vi "YTicks0003.vi"   [LabVIEW 2013]
uses:
  <vilib>/Heliosphere Research LLC/Advanced Plotting Toolkit/api_core/NewPlotType.ctl
  <vilib>/Heliosphere Research LLC/Advanced Plotting Toolkit/Advanced Plotting Toolkit.lvlib
types:
  T1 = typedef "Advanced Plotting Toolkit.lvlib/NewPlotType.ctl" = enum16{"Rectangular Axes", "Polar Axes"}
  T2 = typedef "Advanced Plotting Toolkit.lvlib/PlotID.ctl" = i32
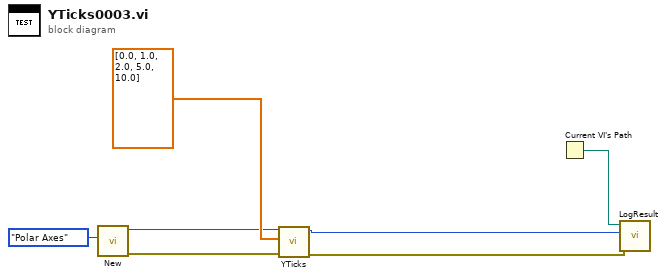
[diagram p0: block diagram]
diagram:
  n1 = call <vilib>:"New.vi"("Plot Type"=NewPlotType."Polar Axes") -> ("error out"=w4:errorcluster, "Plot ID"=w5:T2)  [unwired: 9 in]
  n2 = call <vilib>:"YTicks.vi"("error in (no error)"=w4, "Tick Locations"=dbl[] [0.0, 1.0, 2.0, 5.0, 10.0], "Plot ID"=w5) -> ("error out"=w3:errorcluster, "Plot ID Out"=w2:T2)  [unwired: 7 in]
  n3 = Current VI's Path() -> (path=w7:path)
  n4 = call "LogResult.vi"("Test Result"=w3, "Test Artifact"=w2, "VI Path"=w7) -> ()  [unwired: 9 in]
